vi "Sub Initialize.vi"(8 "error in (no error)":errorcluster, 11 "Measure Object in":refnum<class "Measure Object.lvclass">) -> (0 "error out":errorcluster, 2 "Initialize Result":refnum<class "Acquired Result.lvclass">, 3 "Measure Object out":refnum<class "Measure Object.lvclass">)   [LabVIEW 2015, in "Measure Object.lvclass"]
uses:
  Measure Object.lvclass
  Results/Acquired Result/Acquired Result.lvclass
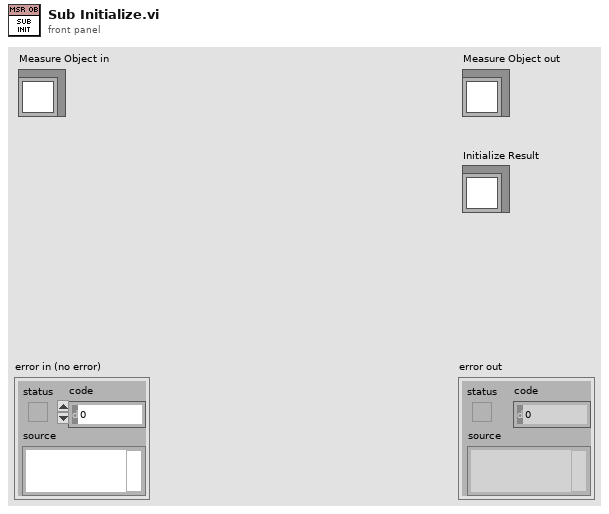
[diagram p1: front panel]
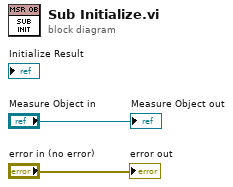
[diagram p0: block diagram]
diagram:
  "error out" <- "error in (no error)"
  "Measure Object out" <- "Measure Object in"
